vi "Clean Set Defaults.vi"(8 "error in (no error)":errorcluster, 11 "VI in":refnum<vi>) -> (0 "error out":errorcluster, 3 "VI":refnum<vi>)   [LabVIEW 2020, in "Conditum-Tools.lvlib" / "Entity Editor.lvclass"]
uses:
  Entity Editor.lvclass
  <vilib>/Utility/traverseref.llb/TRef TravTarget.ctl
  <vilib>/Utility/traverseref.llb/VI Scripting - Traverse.lvlib
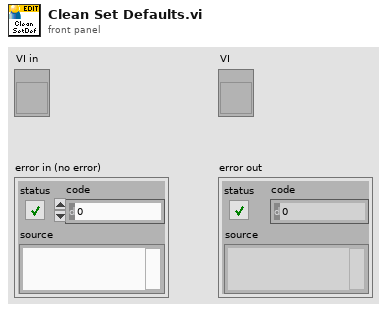
[diagram p1: front panel]
types:
  T1 = typedef "TRef TravTarget.ctl" = enum16{"FP", "BD", "Other"}
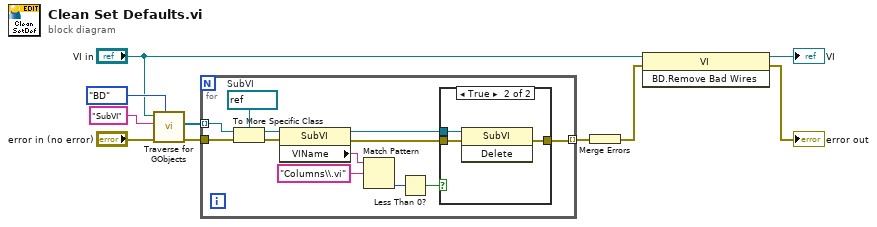
[diagram p0: block diagram]
diagram:
  n1 = call <vilib>:"Traverse for GObjects.vi"("Traverse Target"=TRef_TravTarget."BD", "error in (no error)"="error in (no error)", "Class Name"="SubVI", "VI Refnum"="VI in") -> ("error out"=w5:errorcluster, "References"=w6:refnum<vi>[])  [unwired: 4 in, 2 out]
  n2 = for {
    tunnel: w6 -> [w22] mode=indexing
    tunnel: w5 -> [w19]
    tunnel: [w11] -> w4 mode=indexing
    w20 = refnum<vi> refnum  # SubVI
    n3 = To More Specific Class(target class=w20, reference=w22, error in=w19) -> (specific class reference=w21:refnum<vi>, error out=w18:errorcluster)
    n4 = property class="SubVI"(reference=w21, error in=w18) -> (reference out=w14:refnum<vi>, error out=w13:errorcluster, "VIName"=w17:string)
    n5 = Match Pattern(string=w17, regular expression="Columns\\.vi") -> (offset past match=w15:i32)  [unwired: 1 in, 3 out]
    n6 = Less Than 0?(x=w15) -> (x < 0?=w12:bool)
    n7 = case shown="True" w12 {
      tunnel: w14 -> [_ w26]
      tunnel: w13 -> [w23 w25]
      tunnel: [w23 w24] -> w11
      frame False {
      }
      frame True {
        n8 = invoke class="SubVI" method="Delete"(reference=w26, error in=w25) -> (error out=w24:errorcluster)  [unwired: 1 in, 2 out]
      }
    }
  }
  n9 = Merge Errors(w4) -> (w2:errorcluster)
  n10 = invoke class="VI" method="BD.Remove Bad Wires"(reference="VI in", error in=w2) -> (reference out=→"VI":refnum<vi>, error out=→"error out":errorcluster)  [unwired: 1 in, 1 out]
